vi "rawpower2totalprad.vi"(1 "PowerArray [W]":sgl[][](array[numeric]), 2 "No. of Samples\n[TOA / Sample Rate]":u32=10000, 3 "kbolott_and_volume":dbl[][](array[numeric])) -> (0 "full P_rad [MW]":dbl[](array[numeric]))   [LabVIEW 2014]
panel:
  in  "channel\noffset":i32
  out "constant*geom":dbl
  out "volume":dbl
  out "kbolott":dbl
  out "element after":dbl
  out "volume/kbolott":dbl
  out "element":sgl
  in  "milliseconds to wait":u32
  in  "Nchannels":i32=32
  out "sample array [MW]":dbl[](array[numeric])
  out "constant":dbl
  out "V_Cam":dbl format="%#_13g"
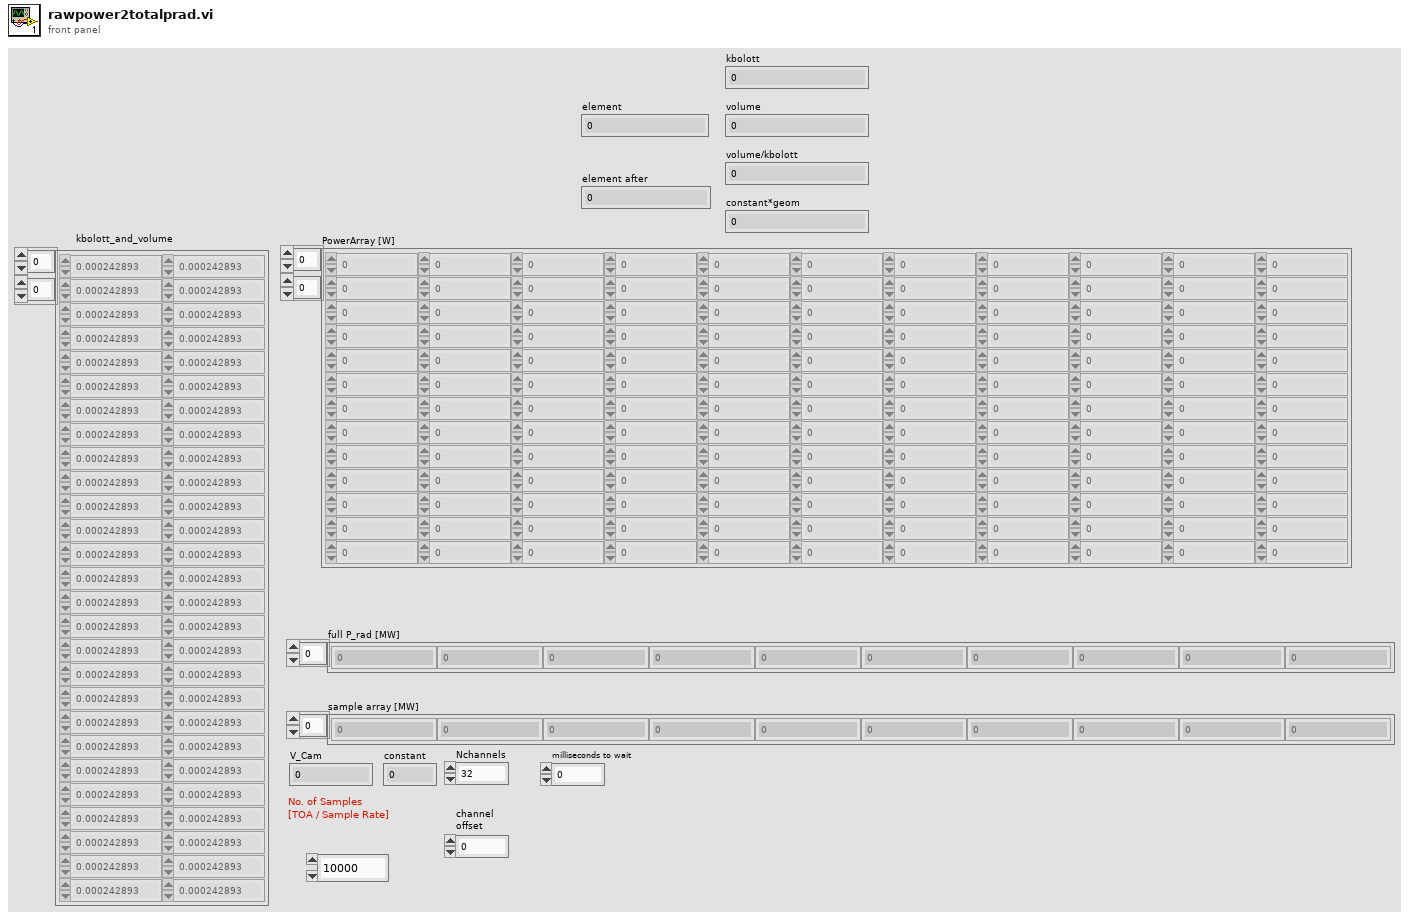
[diagram p1: front panel]
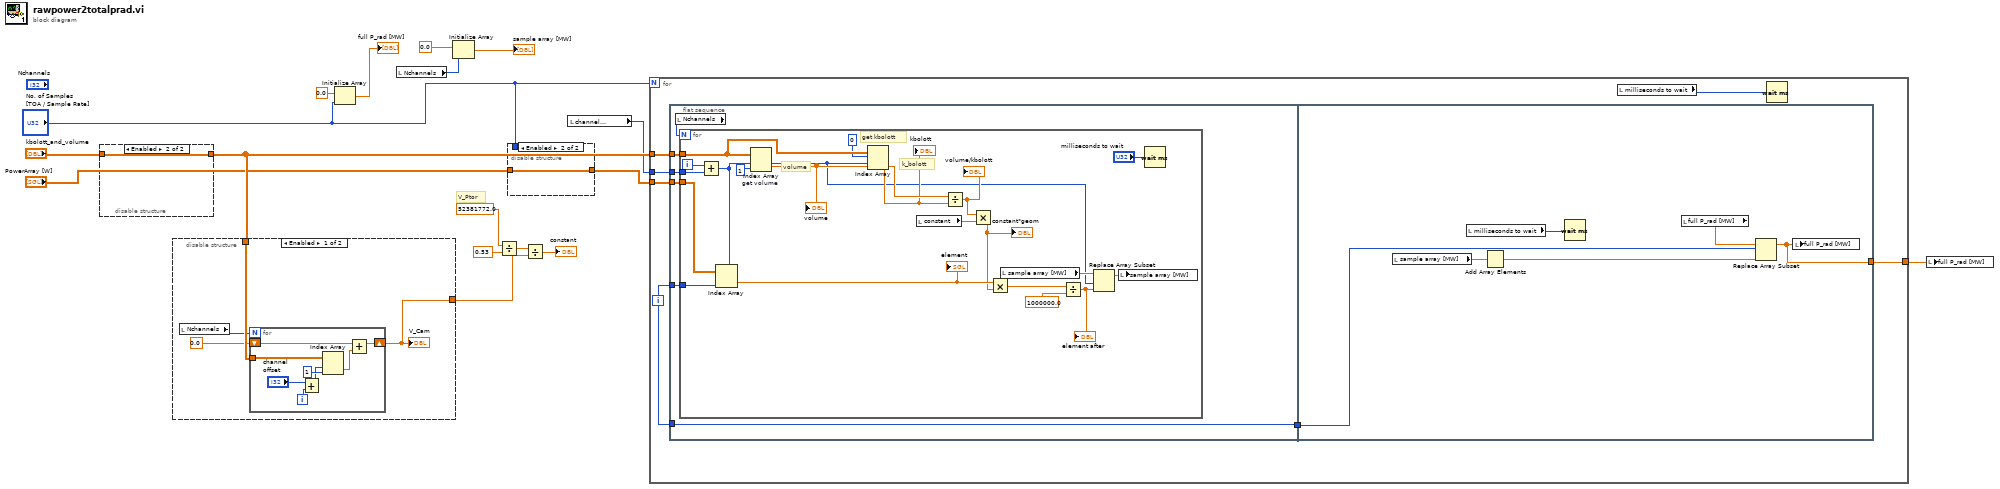
[diagram p0: block diagram]
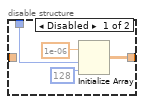
[diagram p2: hidden frame]
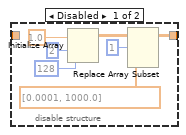
[diagram p3: hidden frame]
diagram:
  # "V_Ptor"
  n1 = disable-structure shown="Enabled" {
    disable-tunnel: [w18 w25] -> w7
    disable-tunnel: "kbolott_and_volume" -> [_ w25]
    frame Disabled {
      n2 = Initialize Array(1.0 ("element"), 2 ("dimension size"), 128 ("dimension size")) -> (w21:dbl[][])
      n3 = Replace Array Subset(array=w21, new element=dbl[] [0.0001, 1000.0] ("new element/subarray"), index (row)=1) -> (w18:dbl[][])  [unwired: 1 in]
    }
    frame Enabled {
    }
  }
  n4 = disable-structure shown="Enabled" {
    disable-tunnel: w7 -> [w29 _]
    disable-tunnel: [w26 _] -> w2
    frame Enabled {
      n5 = local read "Nchannels"() -> (w28:i32)
      n6 = for {
        N: w28 -> [_]
        tunnel: w29 -> [w37]
        shift-right: [w33] -> w26
        shift-left: 0.0 ("V_Cam") -> [w34]
        i -> [w31]
        n7 = Add(x="channel\noffset", y=w31) -> (x+y=w32:i32)
        n8 = Index Array(array=w37, index (row)=w32, index (col)=1 ("disabled index (col)")) -> (element=w36:dbl)
        n9 = Add(x=w34, y=w36) -> (x+y=w33:dbl)
      }
      "V_Cam" <- w26
    }
    frame Disabled {
    }
  }
  n10 = Initialize Array(0.0 ("element"), "No. of Samples\n[TOA / Sample Rate]") -> (→"full P_rad [MW]":dbl[])
  n11 = local read "Nchannels"() -> (w13:i32)
  n12 = Initialize Array(0.0 ("element"), w13) -> (→"sample array [MW]":dbl[])
  n13 = Divide(x=52381772.0, y=0.53) -> (x/y=w11:dbl)
  n14 = disable-structure shown="Enabled" {
    disable-tunnel: "No. of Samples\n[TOA / Sample Rate]" -> [w40 _]
    disable-tunnel: [w38 w42] -> w8
    disable-tunnel: "PowerArray [W]" -> [_ w42]
    frame Disabled {
      n15 = Initialize Array(1e-06 ("element"), w40, 128 ("dimension size")) -> (w38:dbl[][])
    }
    frame Enabled {
    }
  }
  n16 = Divide(x=w11, y=w2) -> (x/y=→"constant":dbl)
  n17 = local read "channel\noffset"() -> (w3:i32)
  n18 = for {
    N: "No. of Samples\n[TOA / Sample Rate]" -> [_]
    tunnel: w8 -> [w49]
    tunnel: w7 -> [w48]
    tunnel: w3 -> [w44]
    tunnel: [w43] -> w1
    i -> [w46]
    n19 = flat-sequence {
      tunnel: w49 -> [w54]
      tunnel: w48 -> [w53]
      tunnel: w46 -> [w52]
      tunnel: [w51] -> w47
      tunnel: w46 -> [w51]
      tunnel: w44 -> [w50]
      tunnel: w47 -> [w80]
      tunnel: [w76] -> w43
      frame #0 {
        n20 = local read "Nchannels"() -> (w55:i32)
        n21 = for {
          N: w55 -> [_]
          tunnel: w54 -> [w72]
          tunnel: w53 -> [w74]
          tunnel: w52 -> [w71]
          tunnel: w50 -> [w56]
          i -> [w58]
          # "get kbolott"
          # "k_bolott"
          # "volume"
          n22 = Add(x=w58, y=w56) -> (x+y=w57:i32)
          n23 = Index Array(array=w72, index (row)=w57, index (col)=w71) -> (element=w68:sgl)
          "element" <- w68
          n24 = Index Array "get volume"(array=w74, index (row)=w57, index (col)=1 ("disabled index (col)")) -> (element=w65:dbl)
          "volume" <- w65
          n25 = Index Array(array=w74, index (row)=w57, index (col)=0 ("disabled index (col)")) -> (element=w59:dbl)
          "kbolott" <- w59
          n26 = local read "constant"() -> (w62:dbl)
          n27 = Divide(x=w65, y=w59) -> (x/y=w64:dbl)
          "volume/kbolott" <- w64
          n28 = Multiply(x=w64, y=w62) -> (x*y=w63:dbl)
          "constant*geom" <- w63
          n29 = Multiply(x=w68, y=w63) -> (x*y=w67:dbl)
          n30 = local read "sample array [MW]"() -> (w61:dbl[])
          n31 = Divide(x=w67, y=1000000.0) -> (x/y=w69:dbl)
          "element after" <- w69
          n32 = Replace Array Subset(array=w61, new element=w69, index=w57) -> (w60:dbl[])
          n33 = local write "sample array [MW]"(w60) -> ()
          n34 = Wait (ms)(milliseconds to wait="milliseconds to wait") -> ()  [unwired: 1 out]
        }
      }
      frame #1 {
        n35 = local read "sample array [MW]"() -> (w77:dbl[])
        n36 = local read "milliseconds to wait"() -> (w79:u32)
        n37 = Add Array Elements(numeric array=w77) -> (sum=w78:dbl)
        n38 = Wait (ms)(milliseconds to wait=w79) -> ()  [unwired: 1 out]
        n39 = local read "full P_rad [MW]"() -> (w81:dbl[])
        n40 = Replace Array Subset(array=w81, new element=w78, index=w80) -> (w76:dbl[])
        n41 = local write "full P_rad [MW]"(w76) -> ()
      }
    }
    n42 = local read "milliseconds to wait"() -> (w45:u32)
    n43 = Wait (ms)(milliseconds to wait=w45) -> ()  [unwired: 1 out]
  }
  n44 = local write "full P_rad [MW]"(w1) -> ()
